vi "Create Dependent Bitfile.vi"(8 "error in (no error)":errorcluster, 11 "Path":path) -> (0 "error out":errorcluster, 3 "OptionalInfo":T1)   [LabVIEW 2014, in "SLSC configuration System Explorer.lvlib"]
uses:
  SLSC configuration System Explorer.lvlib
  <vilib>/NI Veristand/Custom Device API/Dependent File Optional Info.ctl
  Shared/Constants.vi
  <vilib>/NI Veristand/Custom Device API/Custom Device API.lvlib
  Shared/SLSC configuration Shared.lvlib
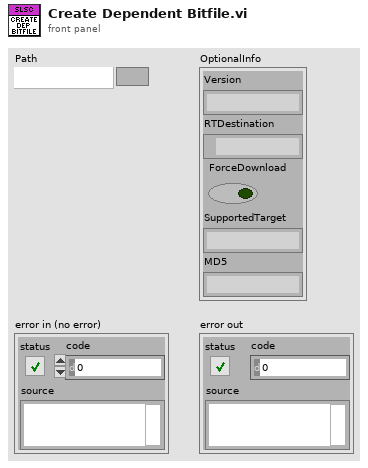
[diagram p1: front panel]
types:
  T1 = typedef "Custom Device API.lvlib/Dependent File Optional Info.ctl" = cluster{"Version":string, "RTDestination":path, "ForceDownload":bool, "SupportedTarget":string, "MD5":string}
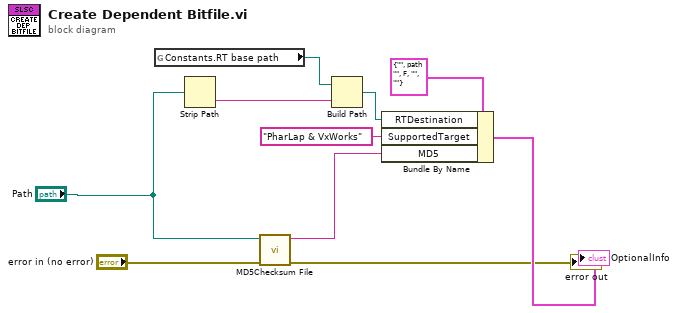
[diagram p0: block diagram]
diagram:
  n1 = global read "Constants.vi" "Constants.RT base path"() -> (w10:path)
  n2 = Strip Path(path="Path") -> (name=w3:string)  [unwired: 1 out]
  n3 = call <vilib>:"MD5Checksum File.vi"("error in (no error)"="error in (no error)", "Path"="Path") -> ("error out"=→"error out":errorcluster, "MD5 message-digest"=w6:string)  [unwired: 8 in]
  n4 = Build Path(base path=w10, name or relative path=w3) -> (appended path=w4:path)
  n5 = Bundle By Name(cluster=T1 {"Version"="", "RTDestination"=path "", "ForceDownload"=FALSE, "SupportedTarget"="", "MD5"=""} ("OptionalInfo"), "RTDestination"=w4, "SupportedTarget"="PharLap & VxWorks", "MD5"=w6) -> (→"OptionalInfo":T1)
